vi "Read fifo config.vi"(8 "error in (no error)":errorcluster, 11 "fifo channel in":refnum<class "fifo channel.lvclass">) -> (0 "error out":errorcluster, 2 "fifo config":T1, 3 "fifo channel out":refnum<class "fifo channel.lvclass">)   [LabVIEW 2017, in "fifo channel.lvclass"]
uses:
  fifo channel.lvclass
  fifo channel settings.ctl
  fifo channel.lvclass/fifo channel.ctl
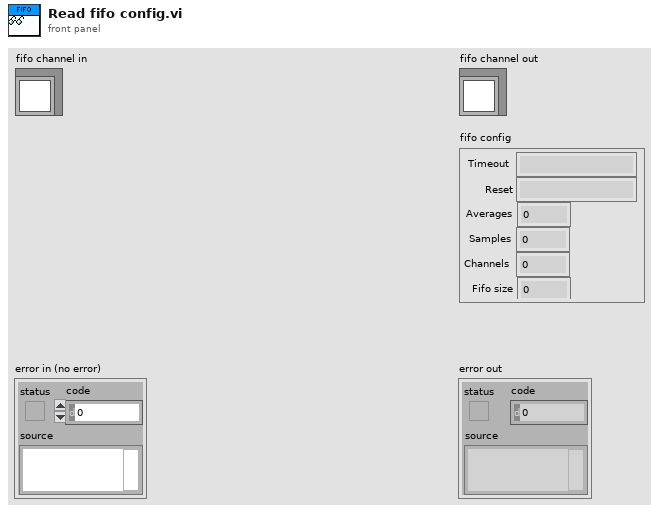
[diagram p1: front panel]
types:
  T1 = typedef "fifo channel.lvclass/fifo channel settings.ctl" = cluster{"Timeout":string, "Reset":string, "Averages":i32, "Samples":u32, "Channels":i32, "Fifo size":u32}
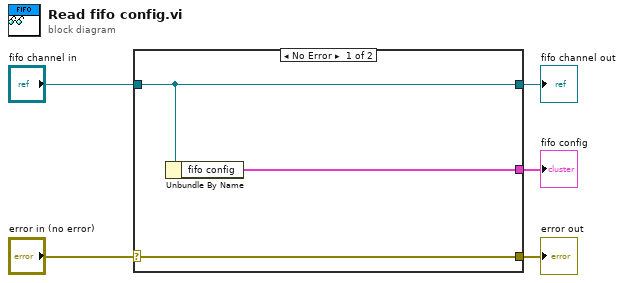
[diagram p0: block diagram]
diagram:
  n1 = case shown="No Error" "error in (no error)" {
    selector: "error in (no error)" -> [w8 w9]
    tunnel: [w8 w9] -> w4
    tunnel: [w7 w10] -> w2
    tunnel: "fifo channel in" -> [w7 w10]
    tunnel: [w6 _] -> w1
    frame No Error {
      n2 = Unbundle By Name(w7) -> ("fifo config"=w6:T1)
    }
    frame Error {
    }
  }
  "error out" <- w4
  "fifo channel out" <- w2
  "fifo config" <- w1
